vi "IDN.vi"(8 "error in (no error)":errorcluster, 11 "RP Communicator in":refnum<class "RP Communicator.lvclass">) -> (0 "error out":errorcluster, 1 "Logic tag":u16, 2 "IDN response":u32=1 format="0x%x (%d)", 3 "RP Communicator out":refnum<class "RP Communicator.lvclass">)   [LabVIEW 2019, in "RP Communicator.lvclass"]
uses:
  RP Communicator.lvclass
  RP Command.ctl
  RP Communicator.lvclass/RP Communicator.ctl
  RP Write Command TCP.vi
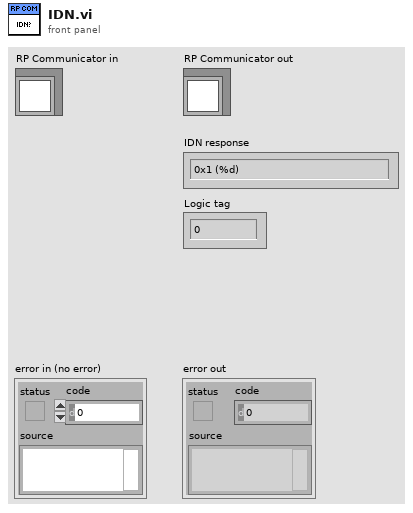
[diagram p1: front panel]
types:
  T1 = enum16{"big-endian, network order", "native, host order", "little-endian"}
  T2 = typedef "RP Command.ctl" = enum16{"Reset", "Read IDN", "Stop server", "Get status", "Get temperature", "Connect client", "Arm", "Software trigger", "Get whole buffer", "Get chunk", "System call", "Get config", "Set config", "Recieve data", "Recieve Calibartion", "Transmit data"}
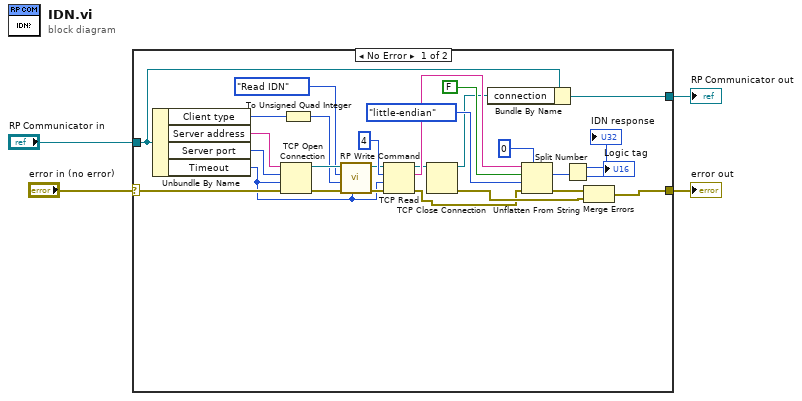
[diagram p0: block diagram]
diagram:
  n1 = case shown="No Error" "error in (no error)" {
    selector: "error in (no error)" -> [w29 w33]
    tunnel: [w10 w33] -> w3
    tunnel: [w24 w32] -> w1
    tunnel: "RP Communicator in" -> [w25 w32]
    frame No Error {
      n2 = Unbundle By Name(w25) -> ("Client type"=w26:enum16{"Control", "Reciever", "Transmitter"}, "Server address"=w31:string, "Server port"=w30:u16, "Timeout"=w5:i32)
      n3 = TCP Open Connection(address=w31, remote port or service name=w30, timeout ms (60000)=w5, error in (no error)=w29) -> (connection ID=w27:refnum<k5>, error out=w28:errorcluster)  [unwired: 1 in]
      n4 = To Unsigned Quad Integer(1:w26) -> (0:w22:u64)
      n5 = call-poly "RP Write Command.vi"("timeout ms (25000)"=w5, "Error In"=w28, "Command payload"=w22, "Command number"=RP_Command."Read IDN", "connection ID"=w27) -> ("Error Out"=w14:errorcluster, "connection ID out"=w15:refnum<k5>)  [unwired: 4 in, 1 out]
      n6 = TCP Read(connection ID=w15, bytes to read=4, error in (no error)=w14, 9:w5) -> (connection ID out=w12:refnum<k5>, data out=w21:string, error out=w8:errorcluster)  [unwired: 1 in]
      n7 = TCP Close Connection(connection ID=w12) -> (connection ID out=w11:refnum<k5>, error out=w9:errorcluster)  [unwired: 2 in]
      n8 = Bundle By Name(cluster=w25, "connection"=w11) -> (w24:refnum<class "RP Communicator.lvclass">)
      n9 = Unflatten From String(type=u32 0, binary string=w21, data includes array or string size? (T)=FALSE, byte order (0:big-endian, network order)=T1."little-endian", error in (no error)=w8) -> (value=w16:u32, error out=w13:errorcluster)  [unwired: 1 out]
      n10 = Split Number(x=w16) -> (hi(x)=→"Logic tag":u16, lo(x)=→"IDN response":u16)
      n11 = Merge Errors(w13, w9) -> (w10:errorcluster)
    }
    frame Error {
    }
  }
  "error out" <- w3
  "RP Communicator out" <- w1
